vi "CRYProbe Window Display.vi"(10 "Row":i32, 11 "Probe Type":string) -> ()   [LabVIEW 2013]
uses:
  <vilib>/Utility/miscctls.llb/LVRectTypeDef.ctl
  CRYWindow/SubVI/CRYMain Sub Window Global.vi
  Global/CRYCurve Library Global.vi
  <vilib>/Utility/inputDevices.llb/mouseAcquire.vi
  <vilib>/Utility/inputDevices.llb/closeMouse.vi
panel:
  in  "Probe Cluster":T1
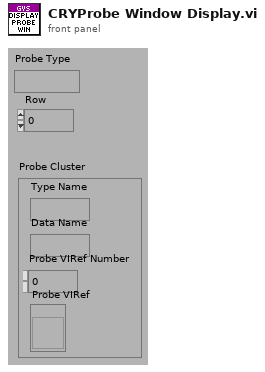
[diagram p1: front panel]
types:
  T1 = cluster{"Type Name":string, "Data Name":string, "Probe VIRef Number":i32, "Probe VIRef":refnum<vi>}
  T2 = enum32{"Invalid", "Standard", "Closed", "Hidden", "Minimized", "Maximized"}
  T3 = typedef "LVRectTypeDef.ctl" = cluster{"Left":i16, "Top":i16, "Right":i16, "Bottom":i16}
  T4 = typedef "CRYData Cluster.ctl" = cluster{"Name":string, "Curve":cluster{"x":dbl, "y":dbl, "z":dbl}[], "X data":u16, "Y data":u16, "Z data":u16, "X axis":u16, "Y axis":u16, "Z axis":u16, "X unit":string, "Y unit":string, "Z unit":string, "X dB ref":dbl, "Y dB ref":dbl, "Z dB ref":dbl, "single val":bool, "protected":bool, "display X":bool, "display Y":bool, "display Z":bool, "Test Info":string, "Step No.":i32, "Plot Settings":cluster{"Color":u32, "Interpolation":u8, "Point Style":u8, "Line Style":u8, "Point Color":u32, "Line Width":u8, "Bar Plot Style":u8, "Fill To":i16}, "AutoProtect":bool}
  T5 = typedef "CRYWaveform Cluster.ctl" = cluster{"Waveform":cluster{"X0":dbl, "dX":dbl, "Y":sgl[]}, "X data":u16, "Y data":u16, "Y axis":u16, "X unit":string, "Y unit":string, "Y dB ref":dbl, "display Y":bool, "display X":bool, "Overload?":bool, "Test Info":string, "Step No.":i32, "Name":string, "protected":bool, "Sqc history":string[], "Signal Channel ID":i32, "Plot Settings":cluster{"Color":u32, "Interpolation":u8, "Point Style":u8, "Line Style":u8, "Point Color":u32, "Line Width":u8, "Bar Plot Style":u8, "Fill To":i16}, "AutoProtect":bool}
  T6 = typedef "CRYResult Cluster.ctl" = cluster{"Name":string, "Margin":dbl, "unit":string, "Verdict":bool, "Limit":string, "Max/Min":string, "protected":bool, "Step No.":i32, "Test Info":string, "AutoProtect":bool}
  T7 = cluster{"Horizontal":i32, "Vertical":i32, "Scrolling":i32}
  T8 = cluster{"Type Name":string, "Data Name":string, "Probe VIRef Number":i32, "Probe VIRef":refnum<vi>}[]
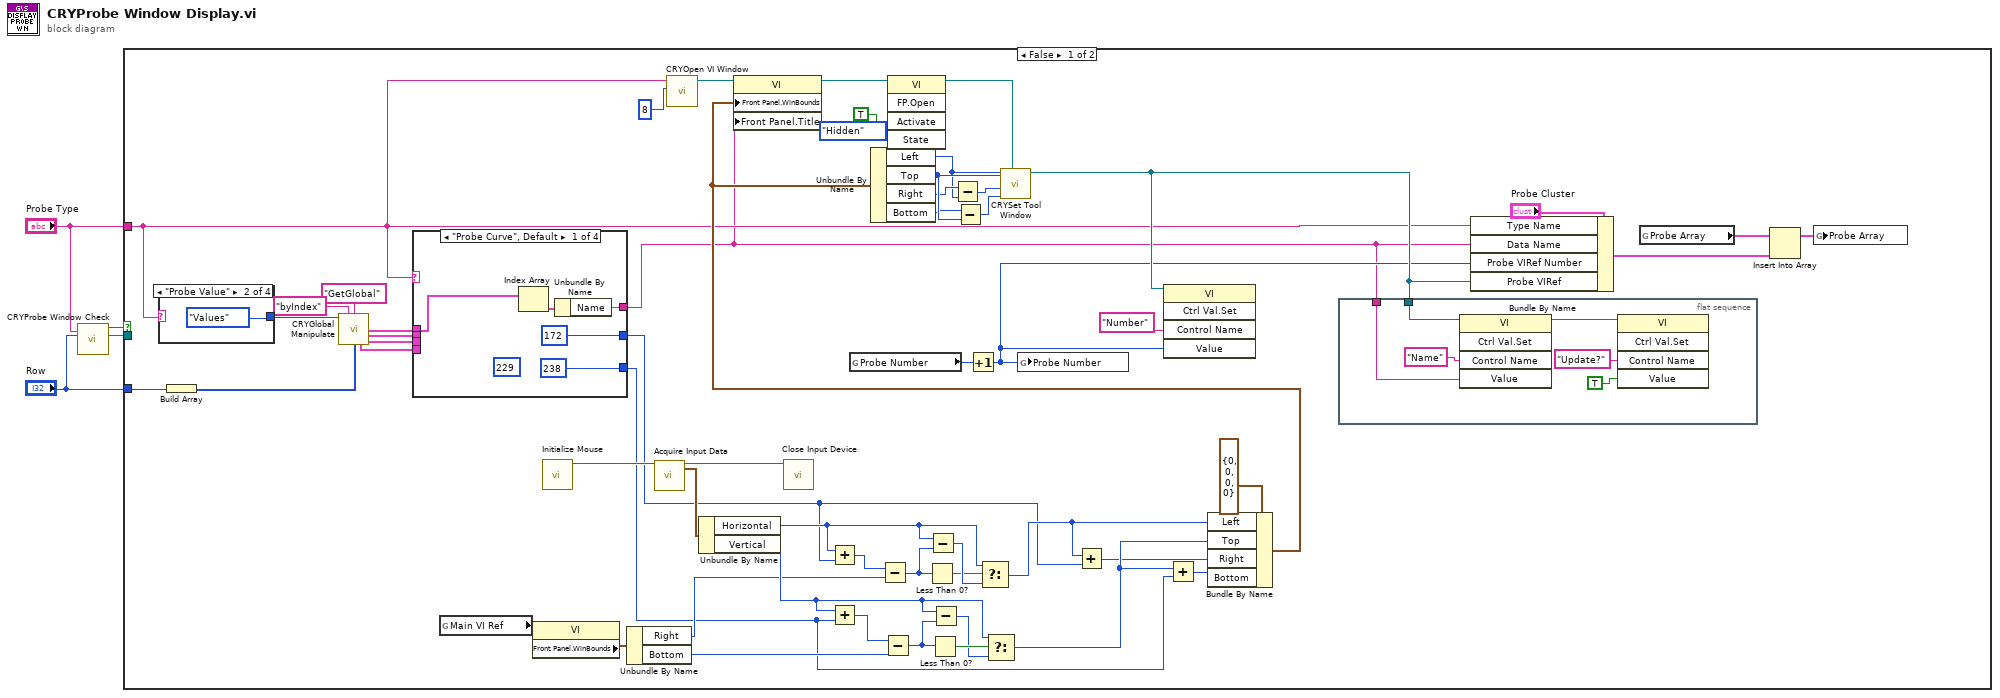
[diagram p0: block diagram]
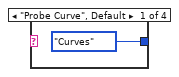
[diagram p2: hidden frame]
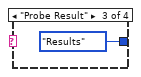
[diagram p3: hidden frame]
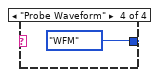
[diagram p4: hidden frame]
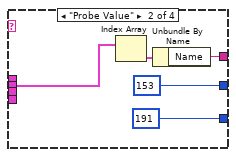
[diagram p5: hidden frame]
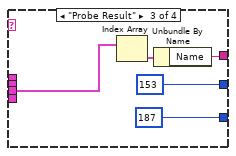
[diagram p6: hidden frame]
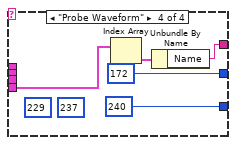
[diagram p7: hidden frame]
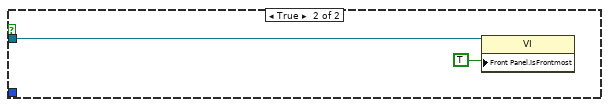
[diagram p8: hidden frame]
diagram:
  n1 = call "CRYProbe Window Check .vi"("Row"="Row", "Probe Type"="Probe Type") -> ("Probe VI Ref"=w1:refnum<vi>, "Exist?"=w2:bool)  [unwired: 8 out]
  n2 = case shown="False" w2 {
    tunnel: "Row" -> [w6 _]
    tunnel: "Probe Type" -> [w15 _]
    tunnel: w1 -> [_ w91]
    frame False {
      n3 = case shown="\"Probe Value\"" w15 {
        tunnel: [enum16{"Curves", "Values", "Results", "WFM"}."Curves" ("Type") enum16{"Curves", "Values", "Results", "WFM"}."Values" ("Type") enum16{"Curves", "Values", "Results", "WFM"}."Results" ("Type") enum16{"Curves", "Values", "Results", "WFM"}."WFM" ("Type")] -> w7
        frame "Probe Curve", Default {
        }
        frame "Probe Value" {
        }
        frame "Probe Result" {
        }
        frame "Probe Waveform" {
        }
      }
      n4 = Build Array(w6) -> (w5:i32[])
      n5 = call "CRYGlobal Manipulate.vi"("Type"=w7, "sOption"="byIndex", "sAction"="GetGlobal", "nData"=w5) -> ("Curves Out"=w12:T4[], "Values Out"=w11:T4[], "WFM Out"=w9:T5[], "Results Out"=w10:T6[])  [unwired: 5 in, 3 out]
      n6 = case shown="\"Probe Curve\", Default" w15 {
        tunnel: [172 ("y") 153 ("y") 153 ("y") 172 ("y")] -> w35
        tunnel: [238 ("y") 191 ("y") 187 ("y") 240 ("y")] -> w36
        tunnel: [w72 w77 w82 w87] -> w8
        tunnel: w12 -> [w71 _ _ _]
        tunnel: w11 -> [_ w76 _ _]
        tunnel: w10 -> [_ _ w81 _]
        tunnel: w9 -> [_ _ _ w86]
        frame "Probe Curve", Default {
          (unwired) 229 ("y")
          n7 = Index Array(array=w71) -> (element=w73:T4)  [unwired: 1 in]
          n8 = Unbundle By Name(w73) -> ("Name"=w72:string)
        }
        frame "Probe Value" {
          n9 = Index Array(array=w76) -> (element=w78:T4)  [unwired: 1 in]
          n10 = Unbundle By Name(w78) -> ("Name"=w77:string)
        }
        frame "Probe Result" {
          n11 = Index Array(array=w81) -> (element=w83:T6)  [unwired: 1 in]
          n12 = Unbundle By Name(w83) -> ("Name"=w82:string)
        }
        frame "Probe Waveform" {
          (unwired) 229 ("y")
          (unwired) 237 ("y")
          n13 = Index Array(array=w86) -> (element=w88:T5)  [unwired: 1 in]
          n14 = Unbundle By Name(w88) -> ("Name"=w87:string)
        }
      }
      n15 = global read "CRYMain Sub Window Global.vi" "Main VI Ref"() -> (w54:refnum<vi>)
      n16 = property class="VI"(reference=w54) -> ("Front Panel.WinBounds"=w53:T3)  [unwired: 1 in, 2 out]
      n17 = call <vilib>:"Initialize Mouse.vi"() -> ("device ID"=w58:refnum<k1>)  [unwired: 1 in, 10 out]
      n18 = Unbundle By Name(w53) -> ("Right"=w41:i16, "Bottom"=w52:i16)
      n19 = call-poly <vilib>:"Acquire Input Data.vi"("device ID"=w58) -> ("device ID"=w57:refnum<k1>, "axis info"=w55:T7)  [unwired: 2 in, 15 out]
      n20 = call "CRYOpen VI Window.vi"("options"=8, "WindowType"=w15) -> ("VI Ref Out"=w59:refnum<vi>)  [unwired: 9 out]
      n21 = Unbundle By Name(w55) -> ("Horizontal"=w39:i32, "Vertical"=w50:i32)
      n22 = call-poly <vilib>:"Close Input Device.vi"("device ID"=w57) -> ()  [unwired: 1 in, 9 out]
      n23 = Add(x=w39, y=w35) -> (x+y=w40:i32)
      n24 = Add(x=w50, y=w36) -> (x+y=w48:i32)
      n25 = global read "CRYCurve Library Global.vi" "Probe Number"() -> (w20:i32)
      n26 = Subtract(x=w40, y=w41) -> (x-y=w44:i32)
      n27 = Subtract(x=w48, y=w52) -> (x-y=w45:i32)
      n28 = Less Than 0?(x=w44) -> (x < 0?=w42:bool)
      n29 = Subtract(x=w39, y=w44) -> (x-y=w43:i32)
      n30 = Less Than 0?(x=w45) -> (x < 0?=w51:bool)
      n31 = Subtract(x=w50, y=w45) -> (x-y=w49:i32)
      n32 = Increment(x=w20) -> (x+1=w16:i32)
      n33 = Select(t=w39, s=w42, f=w43) -> (s? t:f=w38:i32)
      n34 = Select(t=w50, s=w51, f=w49) -> (s? t:f=w47:i32)
      n35 = global write "CRYCurve Library Global.vi" "Probe Number"(w16) -> ()
      n36 = Add(x=w38, y=w35) -> (x+y=w37:i32)
      n37 = Add(x=w47, y=w36) -> (x+y=w46:i32)
      n38 = Bundle By Name(cluster=T3 {"Left"=0, "Top"=0, "Right"=0, "Bottom"=0} ("Front Panel Window:Window Bounds"), "Left"=w38, "Top"=w47, "Right"=w37, "Bottom"=w46) -> (w25:T3)
      n39 = property class="VI"(reference=w59, "Front Panel.WinBounds"=w25, "Front Panel.Title"=w8) -> (reference out=w26:refnum<vi>)  [unwired: 1 in, 1 out]
      n40 = Unbundle By Name(w25) -> ("Left"=w29:i16, "Top"=w33:i16, "Right"=w31:i16, "Bottom"=w30:i16)
      n41 = invoke class="VI" method="FP.Open"(reference=w26, "Activate"=TRUE ("Front Panel Window:Open"), "State"=T2."Hidden") -> (reference out=w24:refnum<vi>)  [unwired: 2 in, 4 out]
      n42 = Subtract(x=w31, y=w29) -> (x-y=w32:i16)
      n43 = Subtract(x=w30, y=w33) -> (x-y=w34:i16)
      n44 = call "CRYSet Tool Window.vi"("VI Ref In"=w24, "Height"=w34, "Width"=w32, "Top"=w33, "Left"=w29) -> ("VI Ref Out"=w18:refnum<vi>)  [unwired: 6 out]
      n45 = invoke class="VI" method="Ctrl Val.Set"(reference=w18, "Control Name"="Number" ("Label Name"), "Value"=w16) -> ()  [unwired: 2 in, 5 out]
      n46 = flat-sequence {
        tunnel: w8 -> [w66]
        tunnel: w18 -> [w70]
        frame #0 {
          n47 = invoke class="VI" method="Ctrl Val.Set"(reference=w70, "Control Name"="Name" ("Label Name"), "Value"=w66) -> (reference out=w65:refnum<vi>)  [unwired: 2 in, 4 out]
          n48 = invoke class="VI" method="Ctrl Val.Set"(reference=w65, "Control Name"="Update?" ("Label Name"), "Value"=TRUE) -> ()  [unwired: 2 in, 5 out]
        }
      }
      n49 = Bundle By Name(cluster="Probe Cluster", "Type Name"=w15, "Data Name"=w8, "Probe VIRef Number"=w16, "Probe VIRef"=w18) -> (w19:T1)
      n50 = global read "CRYCurve Library Global.vi" "Probe Array"() -> (w22:T8)
      n51 = Insert Into Array(array=w22, new element=w19) -> (w23:T8)  [unwired: 1 in]
      n52 = global write "CRYCurve Library Global.vi" "Probe Array"(w23) -> ()
    }
    frame True {
      n53 = property class="VI"(reference=w91, "Front Panel.IsFrontmost"=TRUE ("Front Panel Window:Is Frontmost")) -> ()  [unwired: 1 in, 2 out]
    }
  }
